vi "UI.vi"() -> ()   [LabVIEW 2020]
uses:
  UI/MyTextInput.dll
  UI/MyNumericDisplay.dll
  UI/MyCom.dll
  UI/MySlider.dll
  UI/MyButton.dll
panel:
  out "Bool":bool
  in  "ButtonPanel":refnum<k24>(container)
  in  "SliderPanel":refnum<k24>(container)
  in  "ComboBoxPanel":refnum<k24>(container)
  in  "NumericDisplayPanel":refnum<k24>(container)
  in  "TextInputPanel":refnum<k24>(container)
  in  "TextInputPanel":refnum<k24>(container)
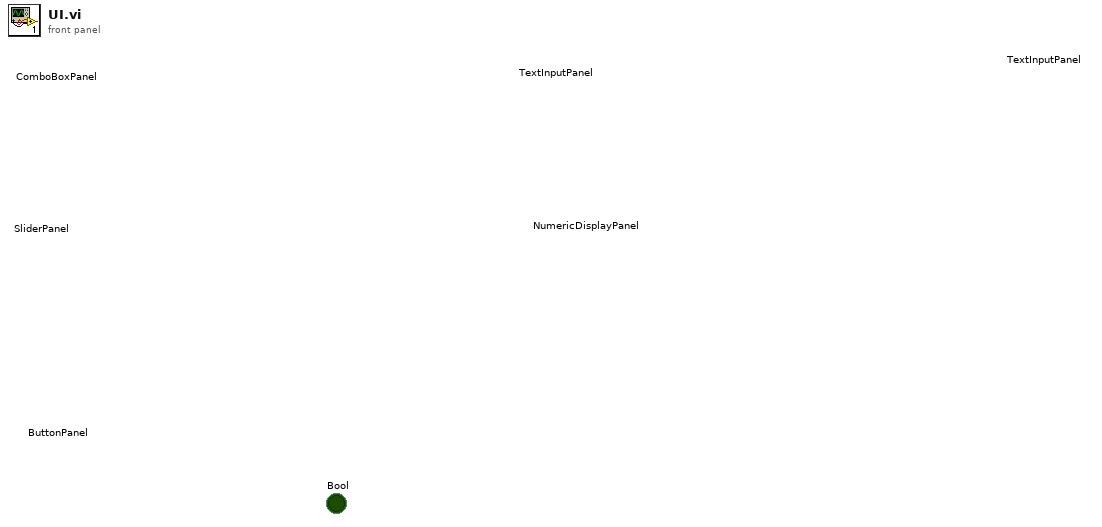
[diagram p1: front panel]
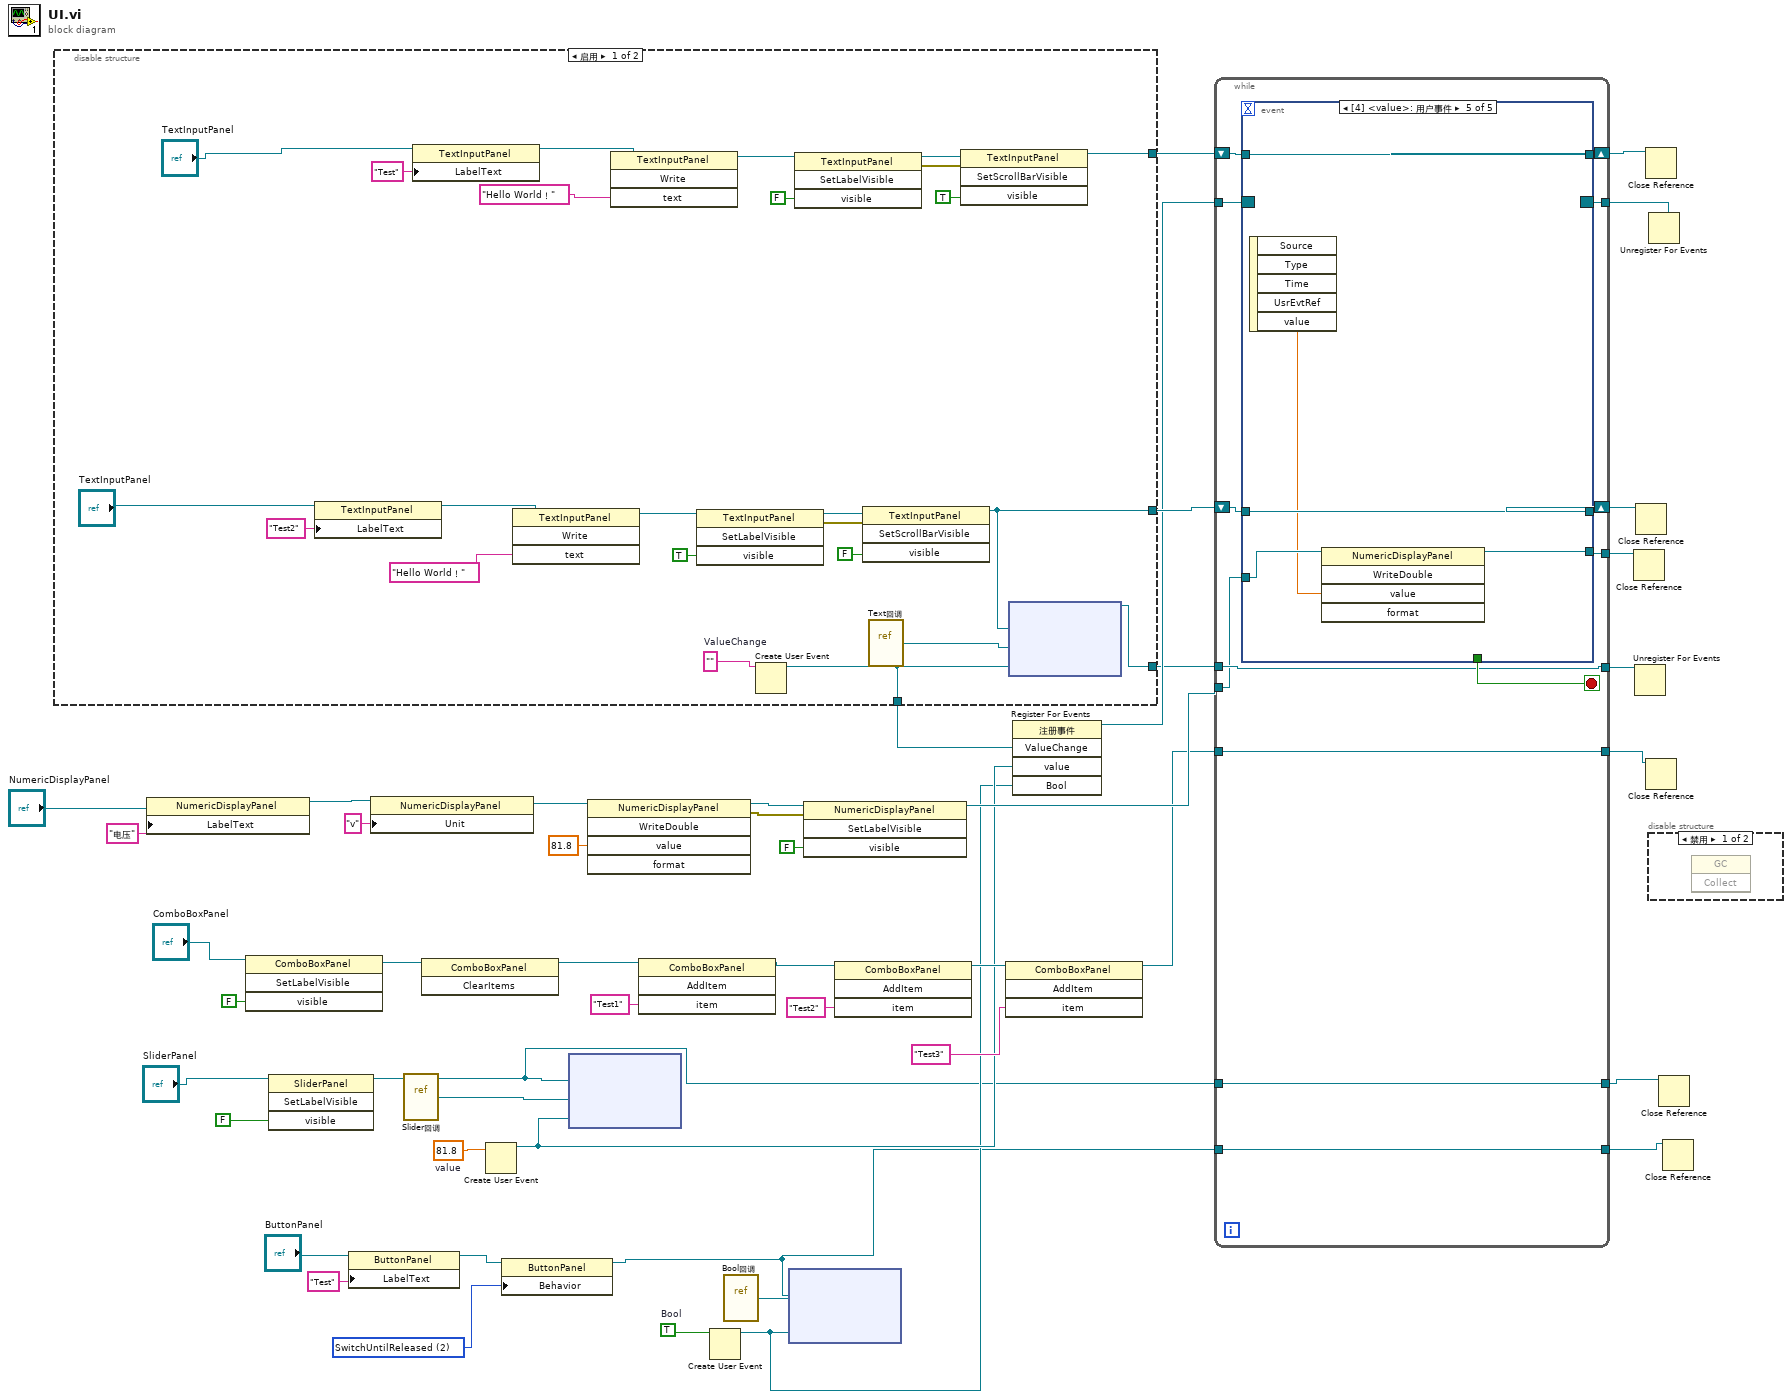
[diagram p0: block diagram]
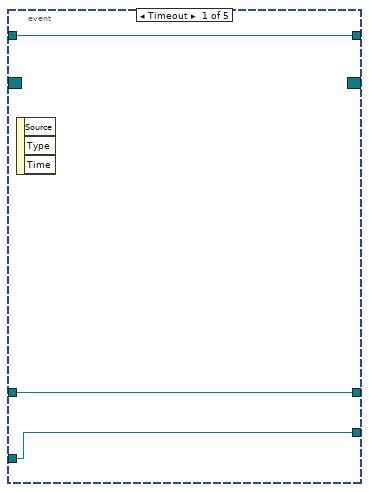
[diagram p3: hidden frame]
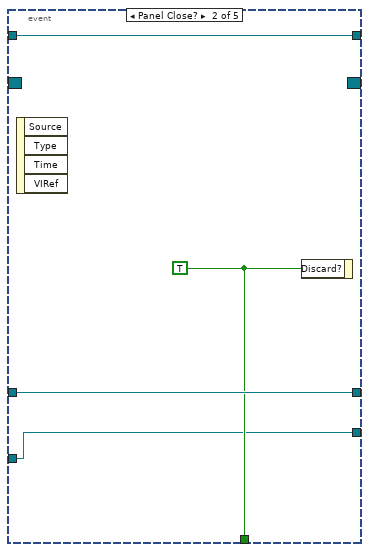
[diagram p4: hidden frame]
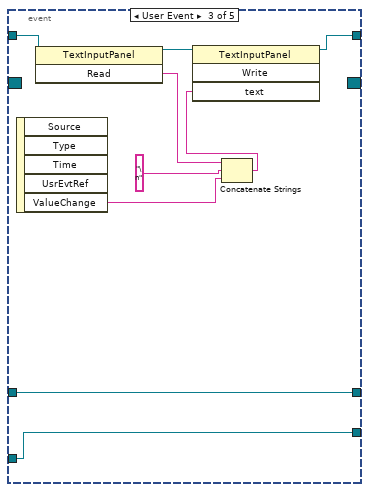
[diagram p5: hidden frame]
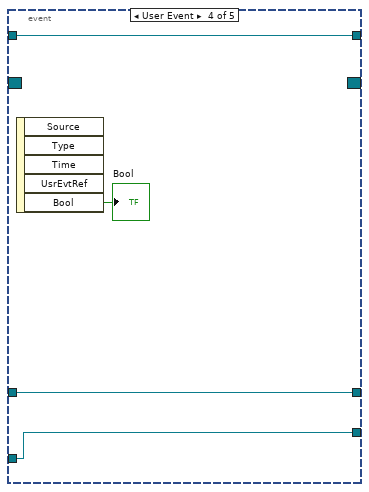
[diagram p6: hidden frame]
diagram:
  w1 = 2 items=["SwitchWhenPressed", "SwitchWhenReleased", "SwitchUntilReleased", "LatchWhenPressed", "LatchWhenReleased"] ("Behavior")
  w8 = TRUE  # Bool
  w16 = 81.8  # value
  n1 = disable-structure shown="启用" {
    disable-tunnel: [w53 _] -> w47
    disable-tunnel: [w52 _] -> w46
    disable-tunnel: [w49 _] -> w43
    disable-tunnel: [w48 _] -> w40
    frame Enabled {
      w51 = ""  # ValueChange
      n2 = property on="属性节点" class="TextInputPanel"(reference="TextInputPanel", "LabelText"="Test2" ("Text")) -> (reference out=w56:refnum<k24>)  [unwired: 1 in, 1 out]
      n3 = property on="属性节点" class="TextInputPanel"(reference="TextInputPanel", "LabelText"="Test" ("Text")) -> (reference out=w70:refnum<k24>)  [unwired: 1 in, 1 out]
      n4 = invoke on="调用节点" class="TextInputPanel" method="Write"(reference=w56, "text"="Hello World！") -> (reference out=w58:refnum<k24>)  [unwired: 2 in, 3 out]
      n5 = invoke on="调用节点" class="TextInputPanel" method="Write"(reference=w70, "text"="Hello World！") -> (reference out=w68:refnum<k24>)  [unwired: 2 in, 3 out]
      n6 = invoke on="调用节点" class="TextInputPanel" method="SetLabelVisible"(reference=w58, "visible"=TRUE) -> (reference out=w60:refnum<k24>, error out=w61:errorcluster)  [unwired: 2 in, 2 out]
      n7 = Create User Event(user event datatype=w51) -> (user event=w49:refnum<user-event>)  [unwired: 1 in, 1 out]
      n8 = invoke on="调用节点" class="TextInputPanel" method="SetLabelVisible"(reference=w68, "visible"=FALSE) -> (reference out=w66:refnum<k24>, error out=w65:errorcluster)  [unwired: 2 in, 2 out]
      n9 = invoke on="调用节点" class="TextInputPanel" method="SetScrollBarVisible"(reference=w60, error in=w61, "visible"=FALSE) -> (reference out=w52:refnum<k24>)  [unwired: 1 in, 3 out]
      n10 = vi-ref "Text回调.vi"() -> ("vi reference"=w50:refnum<vi>)
      n11 = invoke on="调用节点" class="TextInputPanel" method="SetScrollBarVisible"(reference=w66, error in=w65, "visible"=TRUE) -> (reference out=w53:refnum<k24>)  [unwired: 1 in, 3 out]
      n12 = node(w52, w50, w49) -> (w48:refnum<k27>)  [unwired: 2 in, 1 out]
    }
    frame Disabled {
    }
  }
  n13 = property on="属性节点" class="NumericDisplayPanel"(reference="NumericDisplayPanel", "LabelText"="电压") -> (reference out=w37:refnum<k24>)  [unwired: 1 in, 1 out]
  n14 = invoke on="调用节点" class="ComboBoxPanel" method="SetLabelVisible"(reference="ComboBoxPanel", "visible"=FALSE) -> (reference out=w27:refnum<k24>)  [unwired: 2 in, 3 out]
  n15 = invoke on="调用节点" class="SliderPanel" method="SetLabelVisible"(reference="SliderPanel", "visible"=FALSE) -> (reference out=w5:refnum<k24>)  [unwired: 2 in, 3 out]
  n16 = property on="属性节点" class="ButtonPanel"(reference="ButtonPanel", "LabelText"="Test") -> (reference out=w3:refnum<k24>)  [unwired: 1 in, 1 out]
  n17 = property on="属性节点" class="NumericDisplayPanel"(reference=w37, "Unit"="v") -> (reference out=w35:refnum<k24>)  [unwired: 1 in, 1 out]
  n18 = vi-ref "Slider回调.vi"() -> ("vi reference"=w15:refnum<vi>)
  n19 = invoke on="调用节点" class="ComboBoxPanel" method="ClearItems"(reference=w27) -> (reference out=w26:refnum<k24>)  [unwired: 2 in, 2 out]
  n20 = Create User Event(user event datatype=w16) -> (user event=w14:refnum<user-event>)  [unwired: 1 in, 1 out]
  n21 = property on="属性节点" class="ButtonPanel"(reference=w3, "Behavior"=w1) -> (reference out=w2:refnum<k24>)  [unwired: 1 in, 1 out]
  n22 = node(w5, w15, w14) -> ()  [unwired: 2 in, 2 out]
  n23 = invoke on="调用节点" class="NumericDisplayPanel" method="WriteDouble"(reference=w35, "value"=81.8) -> (reference out=w32:refnum<k24>, error out=w33:errorcluster)  [unwired: 3 in, 3 out]
  n24 = invoke on="调用节点" class="ComboBoxPanel" method="AddItem"(reference=w26, "item"="Test1") -> (reference out=w23:refnum<k24>)  [unwired: 2 in, 3 out]
  n25 = Create User Event(user event datatype=w8) -> (user event=w6:refnum<user-event>)  [unwired: 1 in, 1 out]
  n26 = vi-ref "Bool回调.vi"() -> ("vi reference"=w7:refnum<vi>)
  n27 = node(w2, w7, w6) -> ()  [unwired: 2 in, 2 out]
  n28 = invoke on="调用节点" class="NumericDisplayPanel" method="SetLabelVisible"(reference=w32, error in=w33, "visible"=FALSE) -> (reference out=w31:refnum<k24>)  [unwired: 1 in, 3 out]
  n29 = invoke on="调用节点" class="ComboBoxPanel" method="AddItem"(reference=w23, "item"="Test2") -> (reference out=w22:refnum<k24>)  [unwired: 2 in, 3 out]
  n30 = invoke on="调用节点" class="ComboBoxPanel" method="AddItem"(reference=w22, "item"="Test3") -> (reference out=w20:refnum<k24>)  [unwired: 2 in, 3 out]
  n31 = register-events(w43, w14, w6) -> (reference out=w42:refnum<event-registration>)  [unwired: 2 in, 1 out]
  n32 = while {
    tunnel: w42 -> [w80]
    shift-right: [w82] -> w45
    shift-left: w47 -> [w84]
    shift-right: [w81] -> w44
    shift-left: w46 -> [w83]
    tunnel: w40 -> [w78]
    tunnel: [w78] -> w41
    tunnel: w31 -> [w75]
    tunnel: w20 -> [w77]
    tunnel: [w77] -> w19
    tunnel: [w76] -> w13
    tunnel: [w74] -> w12
    tunnel: w2 -> [w73]
    tunnel: [w73] -> w9
    tunnel: w5 -> [w72]
    tunnel: [w72] -> w4
    stop <- w79 stop-if-true
    n33 = event shown="[4] <value>: 用户事件" {
      selector: w80 -> [_ _ _ _ _]
      dyn-events: [_ _ _ _ _] -> w76
      timeout: _ -> [_ _ _ _ _]
      tunnel: w84 -> [w87 w91 w99 w103 w109]
      tunnel: [w87 w91 w93 w103 w109] -> w82
      tunnel: w83 -> [w86 w90 w100 w102 w108]
      tunnel: [w86 w90 w100 w102 w108] -> w81
      tunnel: [_ w89 _ _ _] -> w79
      tunnel: w75 -> [w85 w88 w92 w101 w107]
      tunnel: [w85 w88 w92 w101 w105] -> w74
      event Timeout {
        n34 = event-data() -> ()  [unwired: 1 in, 3 out]
      }
      event Panel Close? {
        w89 = TRUE ("放弃？")
        n35 = event-data() -> ()  [unwired: 1 in, 4 out]
        n36 = event-data("Discard?"=w89) -> ()  [unwired: 1 in, 1 out]
      }
      event User Event {
        n37 = event-data() -> ("ValueChange"=w95:string)  [unwired: 1 in, 4 out]
        n38 = invoke on="调用节点" class="TextInputPanel" method="Read"(reference=w99) -> (reference out=w98:refnum<k24>, "Read"=w97:string)  [unwired: 2 in, 1 out]
        n39 = Concatenate Strings(w97, "\n" ("字符串"), w95) -> (w94:string)
        n40 = invoke on="调用节点" class="TextInputPanel" method="Write"(reference=w98, "text"=w94) -> (reference out=w93:refnum<k24>)  [unwired: 2 in, 3 out]
      }
      event User Event {
        n41 = event-data() -> ("Bool"=→"Bool":bool)  [unwired: 1 in, 4 out]
      }
      event User Event {
        n42 = event-data() -> ("value"=w106:dbl)  [unwired: 1 in, 4 out]
        n43 = invoke on="调用节点" class="NumericDisplayPanel" method="WriteDouble"(reference=w107, "value"=w106) -> (reference out=w105:refnum<k24>)  [unwired: 3 in, 4 out]
      }
    }
  }
  n44 = Close Reference(reference=w12) -> ()  [unwired: 1 in, 1 out]
  n45 = Unregister For Events(event registration refnum=w41) -> ()  [unwired: 1 in, 1 out]
  n46 = Close Reference(reference=w44) -> ()  [unwired: 1 in, 1 out]
  n47 = Close Reference(reference=w45) -> ()  [unwired: 1 in, 1 out]
  n48 = Close Reference(reference=w19) -> ()  [unwired: 1 in, 1 out]
  n49 = Unregister For Events(event registration refnum=w13) -> ()  [unwired: 1 in, 1 out]
  n50 = disable-structure shown="禁用" {
    frame Disabled {
      n51 = invoke on="调用节点" class="GC" method="Collect"() -> ()  [unwired: 3 in, 3 out]
    }
    frame Enabled {
    }
  }
  n52 = Close Reference(reference=w4) -> ()  [unwired: 1 in, 1 out]
  n53 = Close Reference(reference=w9) -> ()  [unwired: 1 in, 1 out]
